vi "FMagMonitor.vi"(2 "error in (no error)":errorcluster, 3 "Max Failed Attempts":i32=5) -> (0 "error out":errorcluster, 1 "FMag Current":dbl)   [LabVIEW 2019]
panel:
  in  "Script Name":string="FMagMonitor"
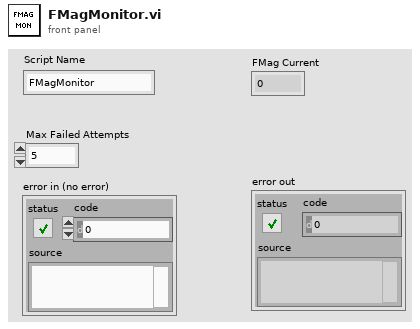
[diagram p1: front panel]
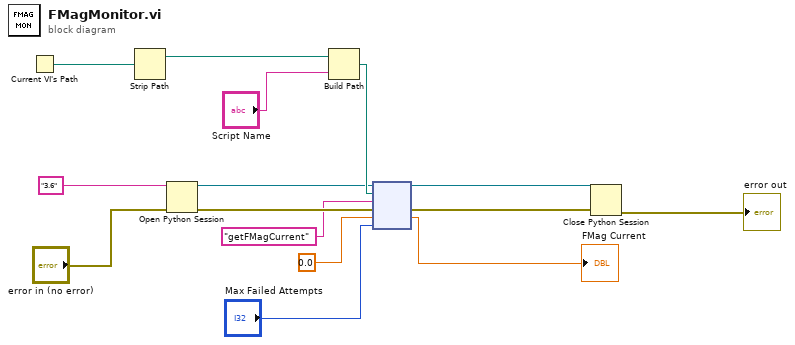
[diagram p0: block diagram]
diagram:
  n1 = Current VI's Path() -> (path=w13:path)
  n2 = Strip Path(path=w13) -> (stripped path=w12:path)  [unwired: 1 out]
  n3 = Open Python Session(python version="3.6" ("Python version"), 3:"error in (no error)") -> (session out=w10:refnum<k35>, error out=w14:errorcluster)  [unwired: 1 in]
  n4 = Build Path(base path=w12, name or relative path="Script Name") -> (appended path=w11:path)
  n5 = node(w10, w11, "getFMagCurrent" ("function name"), w14, 0.0, "Max Failed Attempts") -> (w5:refnum<k35>, w4:errorcluster, →"FMag Current":dbl)  [unwired: 1 in, 2 out]
  n6 = Close Python Session(session in=w5, error in=w4) -> (11:→"error out":errorcluster)
